vi "Is Zombie.vi"(8 "Error In":errorcluster, 11 "GObject In":refnum<vi>) -> (0 "Error Out":errorcluster, 2 "Zombie?":bool, 3 "GObject Out":refnum<vi>)   [LabVIEW 2017, in "Toolkit.lvlib"]
doc: "Checks if a grave has a zombie (enabled corpse frame). A zombie is a Diagram Disable Structure with its legacy code frame (corpse) enabled."
uses:
  Toolkit.lvlib
  Typedefs/Grave Frames.ctl
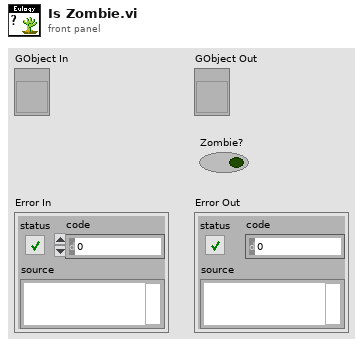
[diagram p1: front panel]
types:
  T1 = typedef "Toolkit.lvlib/Grave Frames.ctl" = enum16{"Corpse", "Spirit"}
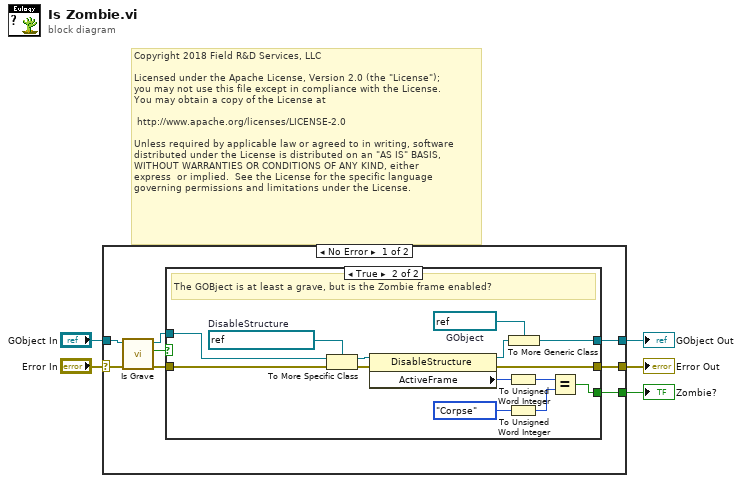
[diagram p0: block diagram]
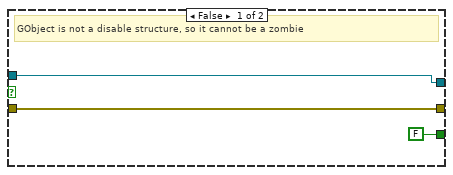
[diagram p2: hidden frame]
diagram:
  # "Copyright 2018 Field R&D Services, LLC\n\nLicensed under the Apache License, Version 2.0 (the \"License\");\nyou may not use this file except in compliance with the License.\nYou may obtain a copy of the License at\n\n\thttp://www.apache.org/licenses/LICENSE-2.0\n\nUnless required by applicable law or agreed to in writing, software\ndistributed under the License is distributed on an \"AS IS\" BASIS,\nWITHOUT WARRANTIES OR CONDITIONS OF ANY KIND, either \nexpress  or implied.  See the License for the specific language \ngoverning permissions and limitations under the License."
  n1 = case shown="No Error" "Error In" {
    selector: "Error In" -> [w6 w31]
    tunnel: [w13 _] -> w5
    tunnel: "GObject In" -> [w12 w32]
    tunnel: [w8 w31] -> w3
    tunnel: [w7 w32] -> w2
    frame No Error {
      n2 = call "Is Grave.vi"("Error In"=w6, "GObject In"=w12) -> ("Error Out"=w10:errorcluster, "Grave?"=w11:bool, "GObject Out"=w9:refnum<vi>)  [unwired: 7 in]
      n3 = case shown="True" w11 {
        tunnel: [FALSE w21] -> w13
        tunnel: w10 -> [w15 w27]
        tunnel: w9 -> [w14 w30]
        tunnel: [w15 w20] -> w8
        tunnel: [w14 w26] -> w7
        frame False {
          # "GObject is not a disable structure, so it cannot be a zombie"
        }
        frame True {
          w25 = refnum<vi> refnum  # GObject
          w28 = refnum<vi> refnum  # DisableStructure
          # "The GOBject is at least a grave, but is the Zombie frame enabled?"
          n4 = To More Specific Class(target class=w28, reference=w30, error in=w27) -> (specific class reference=w29:refnum<vi>, error out=w23:errorcluster)
          n5 = property class="DisableStructure"(reference=w29, error in=w23) -> (reference out=w24:refnum<vi>, error out=w20:errorcluster, "ActiveFrame"=w22:i16)
          n6 = To Unsigned Word Integer(number=w22) -> (unsigned 16bit integer=w19:u16)
          n7 = To Unsigned Word Integer(number=Grave_Frames."Corpse" ("Frame")) -> (unsigned 16bit integer=w17:u16)
          n8 = To More Generic Class(target class=w25, reference=w24) -> (generic class reference=w26:refnum<vi>)
          n9 = Equal?(x=w19, y=w17) -> (x = y?=w21:bool)
        }
      }
    }
    frame Error {
    }
  }
  "Zombie?" <- w5
  "GObject Out" <- w2
  "Error Out" <- w3
